vi "Configure Scale.vi"(0 "VISA resource name":refnum<visa-resource-name>, 1 "Enable Inversion Reading (F: Disable)":bool, 2 "Offset (0)":dbl, 3 "Gain Value (1)":dbl=1.0, 5 "Function Operation (0: Simple NULL Operation)":i32(ring) items=["Simple Null Operation", "Percent Change Operation", "Parts Per Million Operation", "Parts Per Billion Operation", "Mx-B Operation"], 7 "Enable Scaling Function (T: Enable)":bool=TRUE, 9 "Enable Calculate1 (T: Enable)":bool=TRUE, 11 "error in (no error)":errorcluster, 12 "Enable Auto Reference (T: Enable)":bool=TRUE, 13 "Reference (0)":dbl) -> (4 "VISA resource name out":refnum<visa-resource-name>, 15 "error out":errorcluster)   [LabVIEW 2021, in "Agilent 532XX Series.lvlib"]
doc: "Configures the parameters required for function operation."
uses:
  <instrlib>/Agilent 532XX Series/Agilent 532XX Series.lvlib
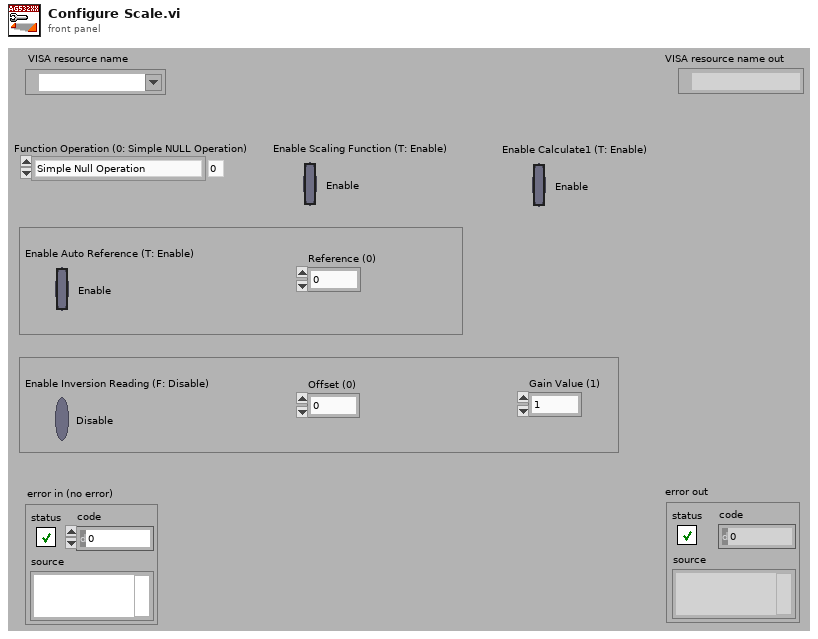
[diagram p1: front panel]
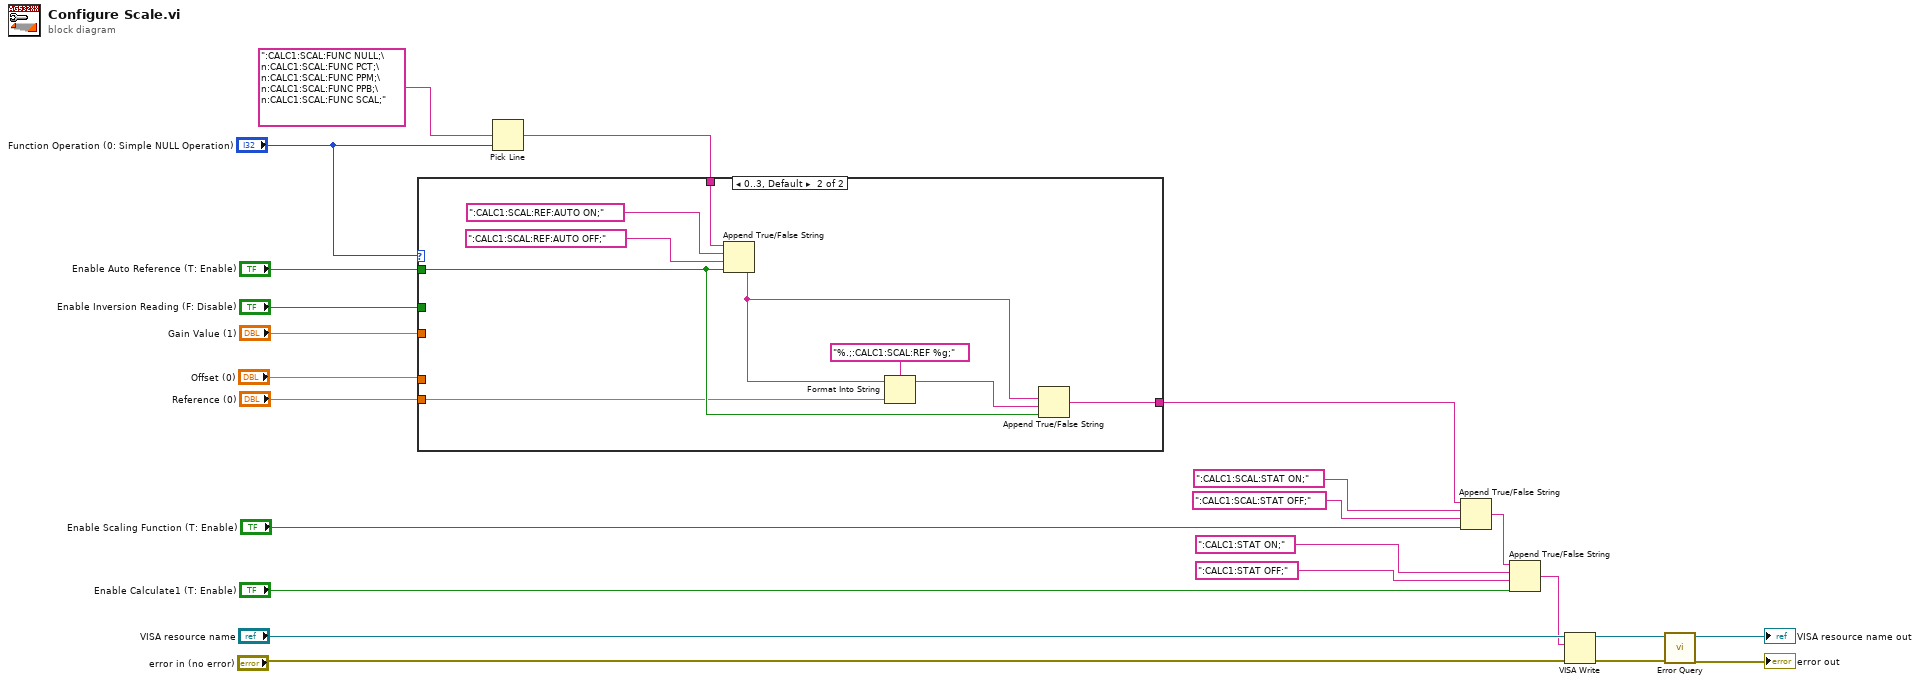
[diagram p0: block diagram]
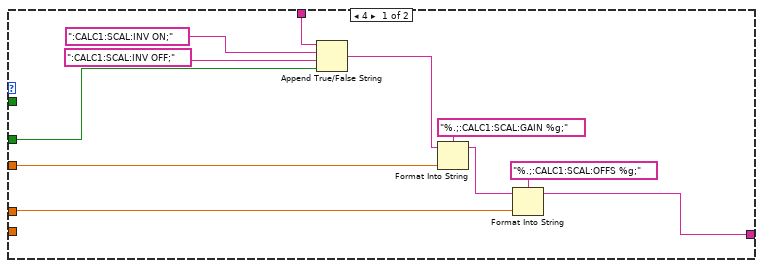
[diagram p2: hidden frame]
diagram:
  n1 = Pick Line(multi-line string=":CALC1:SCAL:FUNC NULL;\n:CALC1:SCAL:FUNC PCT;\n:CALC1:SCAL:FUNC PPM;\n:CALC1:SCAL:FUNC PPB;\n:CALC1:SCAL:FUNC SCAL;", line index="Function Operation (0: Simple NULL Operation)") -> (output string=w12:string)  [unwired: 1 out]
  n2 = case shown="0..3, Default" "Function Operation (0: Simple NULL Operation)" {
    tunnel: w12 -> [w32 w35]
    tunnel: [w31 w41] -> w7
    tunnel: "Enable Auto Reference (T: Enable)" -> [_ w37]
    tunnel: "Reference (0)" -> [_ w36]
    tunnel: "Enable Inversion Reading (F: Disable)" -> [w28 _]
    tunnel: "Gain Value (1)" -> [w26 _]
    tunnel: "Offset (0)" -> [w24 _]
    frame 4 {
      n3 = Append True/False String(1:w28, 2:":CALC1:SCAL:INV OFF;", 3:":CALC1:SCAL:INV ON;", 4:w32) -> (0:w27:string)
      n4 = Format Into String(format string="%.;:CALC1:SCAL:GAIN %g;", initial string=w27, w26) -> (resulting string=w25:string)  [unwired: 1 in, 1 out]
      n5 = Format Into String(format string="%.;:CALC1:SCAL:OFFS %g;", initial string=w25, w24) -> (resulting string=w31:string)  [unwired: 1 in, 1 out]
    }
    frame 0..3, Default {
      n6 = Append True/False String(1:w37, 2:":CALC1:SCAL:REF:AUTO OFF;", 3:":CALC1:SCAL:REF:AUTO ON;", 4:w35) -> (0:w38:string)
      n7 = Format Into String(format string="%.;:CALC1:SCAL:REF %g;", initial string=w38, w36) -> (resulting string=w39:string)  [unwired: 1 in, 1 out]
      n8 = Append True/False String(1:w37, 2:w39, 3:w38) -> (0:w41:string)  [unwired: 1 in]
    }
  }
  n9 = Append True/False String(1:"Enable Scaling Function (T: Enable)", 2:":CALC1:SCAL:STAT OFF;", 3:":CALC1:SCAL:STAT ON;", 4:w7) -> (0:w21:string)
  n10 = Append True/False String(1:"Enable Calculate1 (T: Enable)", 2:":CALC1:STAT OFF;", 3:":CALC1:STAT ON;", 4:w21) -> (0:w6:string)
  n11 = VISA Write(VISA resource name="VISA resource name", write buffer=w6, error in (no error)="error in (no error)") -> (VISA resource name out=w17:refnum<visa-resource-name>, error out=w16:errorcluster)  [unwired: 1 out]
  n12 = call <instrlib>:"Error Query.vi"("error in (no error)"=w16, "VISA resource name"=w17) -> ("error out"=→"error out":errorcluster, "VISA resource name out"=→"VISA resource name out":refnum<visa-resource-name>)  [unwired: 8 out]
